vi "PXIe Health Monitor.vi"() -> ()   [LabVIEW 2018]
doc: "Shows the voltage values, temperature readings, and fan speeds of the Target."
uses:
  <vilib>/nisyscfg/Close (Filter).vi
  <vilib>/nisyscfg/Close (Hardware).vi
  <vilib>/nisyscfg/Close (System).vi
  <vilib>/nisyscfg/nisyscfg.lvlib
  <resource>/objmgr/nicontrollersysapi.rc
  <resource>/objmgr/niflexrioatomicsae.rc
panel:
  out "Temperatures":string[][](table)
  out "Fans":string[][](table)
  out "Voltages":string[][](table)
  in  "User Name":string
  in  "Password":string
  in  "Target (localhost)":refnum<k21>="localhost"
  in  "Stop":bool
  # "Overview: Shows the voltage values, temperature readings, and fan speeds of the Target.\nRequirements:  NI System Configuration, PXI Platform Services\nInstructions:\n1. Select a Target that is connected to a PXIe chassis. Enter User Name and Password if necessary.\n2. Run the VI."
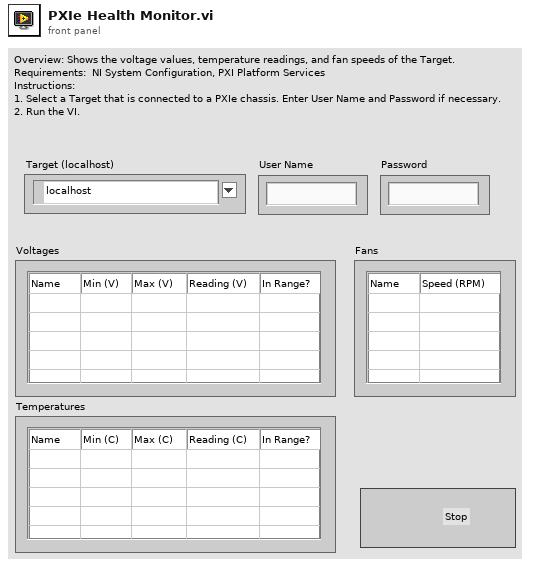
[diagram p1: front panel]
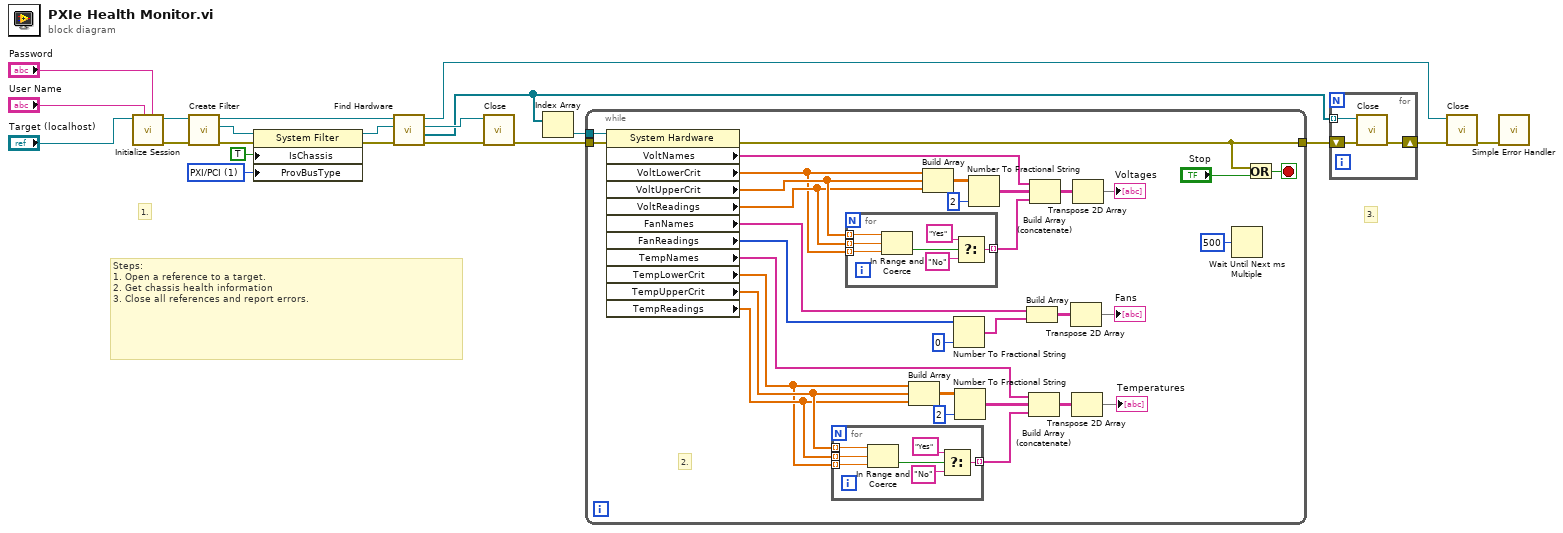
[diagram p0: block diagram]
diagram:
  w10 = u32 1 items=["BuiltIn/System", "PXI/PCI", "USB", "GPIB", "VXI", "Serial", "TCP/IP", "cRIO", "SCXI", "cDAQ", "SwitchBlock", "SCC"] ("Devices & Chassis:Provides Bus Type")
  # "1."
  # "3."
  # "Steps:\n1. Open a reference to a target.\n2. Get chassis health information\n3. Close all references and report errors."
  n1 = call <vilib>:"Initialize Session.vi"("Password"="Password", "User Name"="User Name", "Target (localhost)"="Target (localhost)") -> ("error out"=w8:errorcluster, "Session out"=w9:refnum<k21>)  [unwired: 7 in]
  n2 = call <vilib>:"Create Filter.vi"("error in (no error)"=w8, "Session in"=w9) -> ("error out"=w21:errorcluster, "Filter out"=w18:refnum<k20>, "Session out"=w19:refnum<k21>)  [unwired: 7 in]
  n3 = property class="System Filter"(reference=w18, error in=w21, "IsChassis"=TRUE, "ProvBusType"=w10) -> (reference out=w17:refnum<k20>, error out=w20:errorcluster)
  n4 = call <vilib>:"Find Hardware.vi"("error in (no error)"=w20, "Filter in"=w17, "Session in"=w19) -> ("error out"=w15:errorcluster, "Resources out"=w1:refnum<k20>[], "Filter out"=w16:refnum<k20>, "Session out"=w13:refnum<k21>)  [unwired: 5 in]
  n5 = call-poly <vilib>:"Close.vi"("error in (no error)"=w15, "Filter in"=w16) -> ("error out"=w12:errorcluster)  [unwired: 9 in]
  n6 = Index Array(array=w1) -> (element=w2:refnum<k20>)  [unwired: 1 in]
  n7 = while {
    tunnel: [w49] -> w6
    tunnel: w12 -> [w53]
    tunnel: w2 -> [w48]
    stop <- w51 stop-if-true
    # "2."
    n8 = property class="System Hardware"(reference=w48, error in=w53) -> (error out=w49:errorcluster, "VoltNames"=w45:string[], "VoltLowerCrit"=w40:dbl[], "VoltUpperCrit"=w42:dbl[], "VoltReadings"=w41:dbl[], "FanNames"=w36:string[], "FanReadings"=w35:u32[], "TempNames"=w24:string[], "TempLowerCrit"=w23:dbl[], "TempUpperCrit"=w27:dbl[], "TempReadings"=w26:dbl[])  [unwired: 1 out]
    n9 = for {
      tunnel: [w57] -> w30 mode=indexing
      tunnel: w27 -> [w56] mode=indexing
      tunnel: w26 -> [w55] mode=indexing
      tunnel: w23 -> [w54] mode=indexing
      n10 = In Range and Coerce(upper limit=w56, x=w55, lower limit=w54) -> (In Range?=w60:bool)  [unwired: 1 out]
      n11 = Select(t="Yes", s=w60, f="No") -> (s? t:f=w57:string)
    }
    n12 = for {
      tunnel: w42 -> [w67] mode=indexing
      tunnel: w41 -> [w66] mode=indexing
      tunnel: w40 -> [w65] mode=indexing
      tunnel: [w61] -> w39 mode=indexing
      n13 = In Range and Coerce(upper limit=w67, x=w66, lower limit=w65) -> (In Range?=w64:bool)  [unwired: 1 out]
      n14 = Select(t="Yes", s=w64, f="No") -> (s? t:f=w61:string)
    }
    n15 = Build Array(w23, w27, w26) -> (w25:dbl[][])
    n16 = Build Array(w40, w42, w41) -> (w47:dbl[][])
    n17 = Number To Fractional String(number=w35, precision (6)=i16 0) -> (F-format string=w34:string[])  [unwired: 2 in]
    n18 = Number To Fractional String(number=w25, precision (6)=i16 2) -> (F-format string=w28:string[][])  [unwired: 2 in]
    n19 = Number To Fractional String(number=w47, precision (6)=i16 2) -> (F-format string=w46:string[][])  [unwired: 2 in]
    n20 = Build Array(w36, w34) -> (w33:string[][])
    n21 = Build Array (concatenate)(w24, w28, w30) -> (w29:string[][])
    n22 = Build Array (concatenate)(w45, w46, w39) -> (w44:string[][])
    n23 = Transpose 2D Array(2D array=w33) -> (transposed array=→"Fans":string[][])
    n24 = Transpose 2D Array(2D array=w29) -> (transposed array=→"Temperatures":string[][])
    n25 = Transpose 2D Array(2D array=w44) -> (transposed array=→"Voltages":string[][])
    n26 = Wait Until Next ms Multiple(millisecond multiple=u32 500 ("Wait (ms)")) -> ()  [unwired: 1 out]
    n27 = Or(x=w49, y="Stop") -> (x .or. y?=w51:bool)
  }
  n28 = for {
    shift-right: [w70] -> w7
    shift-left: w6 -> [w69]
    tunnel: w1 -> [w68] mode=indexing
    n29 = call-poly <vilib>:"Close.vi"("error in (no error)"=w69, "Resource in"=w68) -> ("error out"=w70:errorcluster)  [unwired: 9 in]
  }
  n30 = call-poly <vilib>:"Close.vi"("error in (no error)"=w7, "Session in"=w13) -> ("error out"=w11:errorcluster)  [unwired: 9 in]
  n31 = call <vilib>:"Simple Error Handler.vi"("error in (no error)"=w11) -> ()  [unwired: 4 in, 5 out]
